vi "FGV - event exit.vi"(7 "Action (Read)":enum16{"Init", "Read", "Générer", "Supprimer"}(ring)=enum."Read", 8 "entrée d'erreur (pas d'erreur)":errorcluster) -> (0 "sortie d'erreur":errorcluster, 3 "Refnum d'abonnement à des événements":refnum<event-registration>)   [LabVIEW 2019]
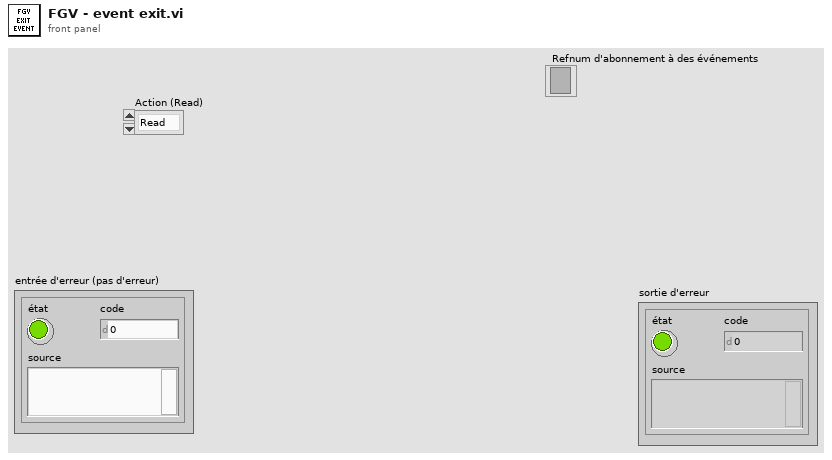
[diagram p1: front panel]
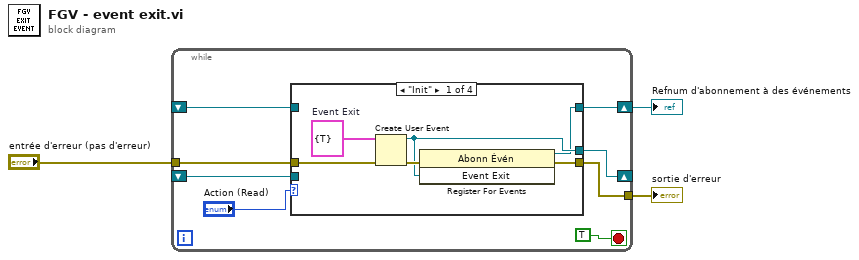
[diagram p0: block diagram]
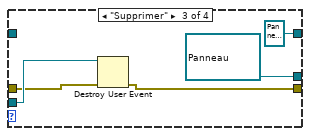
[diagram p3: hidden frame]
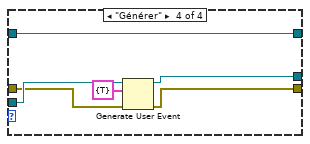
[diagram p4: hidden frame]
diagram:
  n1 = while {
    shift-right: [w9] -> w1
    shift-left: _ -> [w8]
    shift-right: [w10] -> _
    shift-left: _ -> [w7]
    tunnel: "entrée d'erreur (pas d'erreur)" -> [w5]
    tunnel: [w4] -> w2
    stop <- TRUE stop-if-true
    n2 = case shown="\"Init\"" "Action (Read)" {
      tunnel: [w15 w19 refnum<user-event> refnum ("Event Exit") w26] -> w10
      tunnel: [w14 w20 refnum<event-registration> refnum ("Refnum d'abonnement à des événements") w27] -> w9
      tunnel: w8 -> [_ w20 _ w27]
      tunnel: w7 -> [_ w19 w25 w31]
      tunnel: w5 -> [w13 w18 w24 w29]
      tunnel: [w12 w18 w23 w28] -> w4
      frame "Init" {
        w17 = cluster{"Exit?":bool} {"Exit?"=TRUE}  # Event Exit
        n3 = Create User Event(user event datatype=w17, error in=w13) -> (user event=w15:refnum<user-event>, error out=w16:errorcluster)
        n4 = register-events(error in=w16, w15) -> (reference out=w14:refnum<event-registration>, error out=w12:errorcluster)  [unwired: 1 in]
      }
      frame "Read", Default {
      }
      frame "Supprimer" {
        n5 = Destroy User Event(user event=w25, error in=w24) -> (error out=w23:errorcluster)
      }
      frame "Générer" {
        n6 = Generate User Event(user event=w31, event data cluster=cluster{"Exit?":bool} {"Exit?"=TRUE} ("données d'événement"), error in=w29) -> (user event out=w26:refnum<user-event>, error out=w28:errorcluster)  [unwired: 1 in]
      }
    }
  }
  "sortie d'erreur" <- w2
  "Refnum d'abonnement à des événements" <- w1
